vi "Read From Spreadsheet File (I64)-Mod.vi"(0 "file path (dialog if empty)":path, 1 "format (%d)":string="%d", 5 "number of rows (all:-1)":i32=-1, 7 "max characters/row  (no limit:0)":i32, 9 "start of read offset (chars.:0)":i32, 11 "error in":errorcluster, 12 "transpose (no:F)":bool, 14 "delimiter (\\t)":string="\t") -> (3 "new file path (Not A Path if cancelled)":path, 4 "all rows":i64[][](array[numeric]), 6 "first row":i64[](array[numeric]), 8 "EOF?":bool, 10 "mark after read (chars.)":i32, 15 "error out":errorcluster)   [LabVIEW 2017]
doc: "Reads a specified number of lines or rows from a numeric text file beginning at a specified character offset and converts the data to a 2D, double-precision array of numbers, strings, or integers. You must manually select the polymorphic instance you want to use."
panel:
  in  "type (empty)":i64[][](array[numeric])
  # "row\ncolumn"
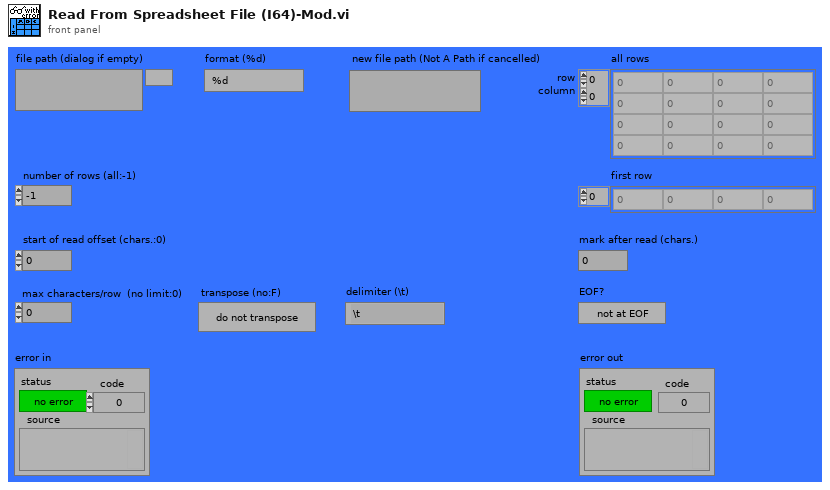
[diagram p1: front panel]
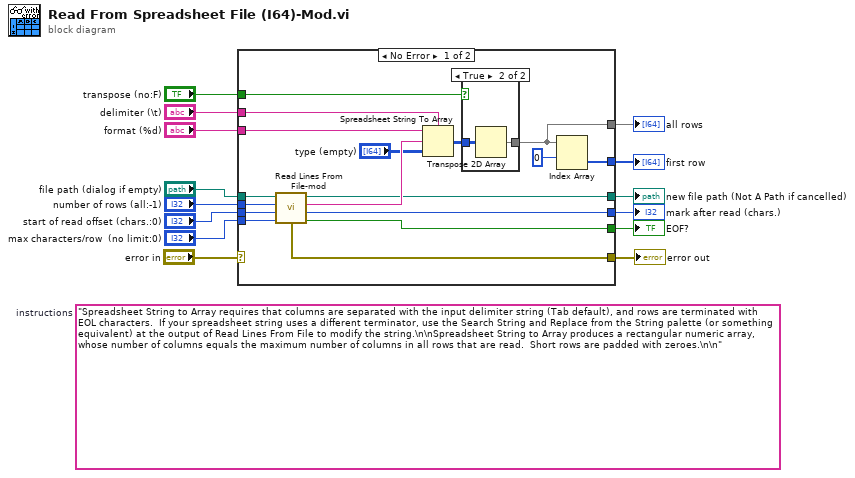
[diagram p0: block diagram]
diagram:
  (unwired) "Spreadsheet String to Array requires that columns are separated with the input delimiter string (Tab default), and rows are terminated with EOL characters.  If your spreadsheet string uses a different terminator, use the Search String and Replace from the String palette (or something equivalent) at the output of Read Lines From File to modify the string.\n\nSpreadsheet String to Array produces a rectangular numeric array, whose number of columns equals the maximum number of columns in all rows that are read.  Short rows are padded with zeroes.\n\n"  # instructions
  n1 = case shown="No Error" "error in" {
    selector: "error in" -> [_ w36]
    tunnel: "number of rows (all:-1)" -> [w31 _]
    tunnel: "file path (dialog if empty)" -> [w30 w35]
    tunnel: "max characters/row  (no limit:0)" -> [w29 _]
    tunnel: "start of read offset (chars.:0)" -> [w28 _]
    tunnel: "transpose (no:F)" -> [w26 _]
    tunnel: [w24 w35] -> w9
    tunnel: [w22 _] -> w8
    tunnel: [w21 _] -> w7
    tunnel: [w20 _] -> w6
    tunnel: "format (%d)" -> [w18 _]
    tunnel: "delimiter (\\t)" -> [w17 _]
    tunnel: [w16 _] -> w3
    tunnel: [w15 w36] -> w2
    frame No Error {
      n2 = call "Read Lines From File-mod.vi"("file path (dialog if empty)"=w30, "number of lines (all:-1)"=w31, "start of read offset (chars.:0)"=w28, "[max characters per line]  (no limit:0)"=w29) -> ("new file path (Not A Path if cancelled)"=w24:path, "line string"=w27:string, "mark after read (chars.)"=w20:i32, "EOF?"=w16:bool, "error out"=w15:errorcluster)  [unwired: 1 in]
      n3 = Spreadsheet String To Array(delimiter (Tab)=w17, format string=w18, spreadsheet string=w27, array type (2D Dbl)="type (empty)") -> (array=w25:i64[][])
      n4 = case shown="True" w26 {
        tunnel: [w32 w34] -> w22
        tunnel: w25 -> [w32 w33]
        frame False {
        }
        frame True {
          n5 = Transpose 2D Array(2D array=w33) -> (transposed array=w34:i64[][])
        }
      }
      n6 = Index Array(array=w22, index (row)=0) -> (element=w21:i64[])  [unwired: 1 in]
    }
    frame Error {
    }
  }
  "new file path (Not A Path if cancelled)" <- w9
  "first row" <- w7
  "mark after read (chars.)" <- w6
  "all rows" <- w8
  "EOF?" <- w3
  "error out" <- w2
